vi "DataBuffer_NET-rebuild.VI"() -> ()   [LabVIEW 2016]
uses:
  C:/Program Files/Ocean Optics/OmniDriver/OOI_HOME/NETOmniDriver-NET20.dll
  Program Files/Ocean Optics/OmniDriver/OOI_HOME/NETOmniDriver-NET20.dll
panel:
  out "getBufferCapacity":i32
  out "isFeatureSupportedDataBuffer":i16
  in  "setBufferCapacity":i32
  in  "spectrometerIndex":i32
  out "Spectrometer Name:":string
  out "Serial Number:":string
  in  "Scans to Average":i32=1 min=1 max=50 step=1
  in  "Boxcar Width":i32=5 min=0 max=50 step=1
  in  "Int. Time (microsec)":i32=100000 min=3000 max=65000000
  out "Number of Spectrometers":i32
  in  "stop":bool
  out "Current Spectrum":cluster{"Y":dbl[], "Y":dbl[]}[](graph)
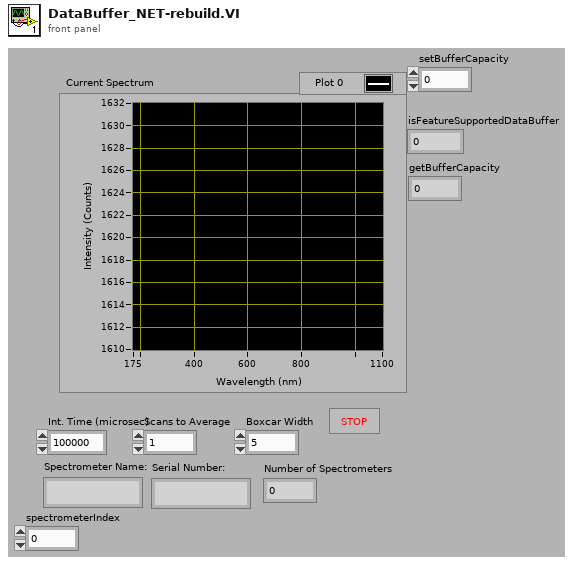
[diagram p1: front panel]
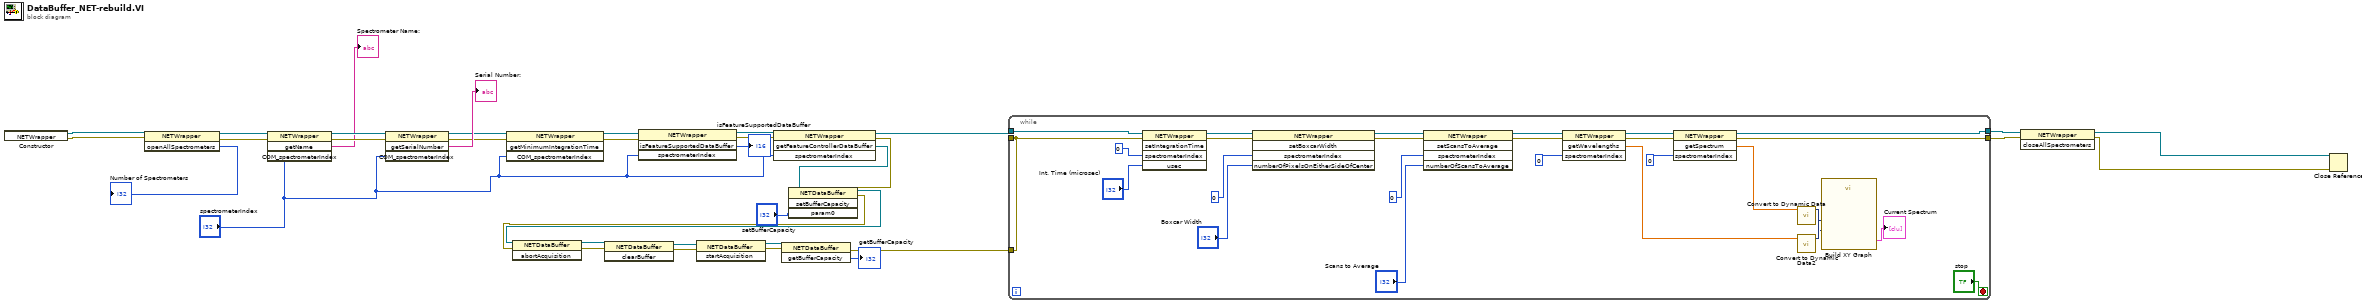
[diagram p0: block diagram]
diagram:
  n1 = constructor class="NETWrapper"() -> (reference out=w23:refnum<k24>, error out=w22:errorcluster)  [unwired: 3 in, 1 out]
  n2 = invoke class="NETWrapper" method="openAllSpectrometers"(reference=w23, error in=w22) -> (reference out=w31:refnum<k24>, error out=w30:errorcluster, "openAllSpectrometers"=→"Number of Spectrometers":i32)  [unwired: 1 in]
  n3 = invoke class="NETWrapper" method="getName"(reference=w31, error in=w30, "COM_spectrometerIndex"="spectrometerIndex") -> (reference out=w29:refnum<k24>, error out=w28:errorcluster, "getName"=→"Spectrometer Name:":string)  [unwired: 1 in, 1 out]
  n4 = invoke class="NETWrapper" method="getSerialNumber"(reference=w29, error in=w28, "COM_spectrometerIndex"="spectrometerIndex") -> (reference out=w26:refnum<k24>, error out=w25:errorcluster, "getSerialNumber"=→"Serial Number:":string)  [unwired: 1 in, 1 out]
  n5 = invoke class="NETWrapper" method="getMinimumIntegrationTime"(reference=w26, error in=w25, "COM_spectrometerIndex"="spectrometerIndex") -> (reference out=w21:refnum<k24>, error out=w20:errorcluster)  [unwired: 1 in, 2 out]
  n6 = invoke class="NETWrapper" method="isFeatureSupportedDataBuffer"(reference=w21, error in=w20, "spectrometerIndex"="spectrometerIndex") -> (reference out=w19:refnum<k24>, error out=w18:errorcluster, "isFeatureSupportedDataBuffer"=→"isFeatureSupportedDataBuffer":i16)  [unwired: 1 in, 1 out]
  n7 = invoke class="NETWrapper" method="getFeatureControllerDataBuffer"(reference=w19, error in=w18, "spectrometerIndex"="spectrometerIndex") -> (reference out=w17:refnum<k24>, error out=w9:errorcluster, "getFeatureControllerDataBuffer"=w11:refnum<k24>)  [unwired: 1 in, 1 out]
  n8 = invoke class="NETDataBuffer" method="setBufferCapacity"(reference=w11, error in=w9, "param0"="setBufferCapacity") -> (reference out=w10:refnum<k24>, error out=w7:errorcluster)  [unwired: 1 in, 2 out]
  n9 = invoke class="NETDataBuffer" method="abortAcquisition"(reference=w10, error in=w7) -> (reference out=w15:refnum<k24>, error out=w14:errorcluster)  [unwired: 1 in, 1 out]
  n10 = invoke class="NETDataBuffer" method="clearBuffer"(reference=w15, error in=w14) -> (reference out=w13:refnum<k24>, error out=w12:errorcluster)  [unwired: 1 in, 1 out]
  n11 = invoke class="NETDataBuffer" method="startAcquisition"(reference=w13, error in=w12) -> (reference out=w5:refnum<k24>, error out=w4:errorcluster)  [unwired: 1 in, 1 out]
  n12 = invoke class="NETDataBuffer" method="getBufferCapacity"(reference=w5, error in=w4) -> (error out=w8:errorcluster, "getBufferCapacity"=→"getBufferCapacity":i32)  [unwired: 1 in, 1 out]
  n13 = while {
    tunnel: [w58] -> w35
    tunnel: [w57] -> w34
    tunnel: w17 -> [w50]
    tunnel: [w36] -> _
    tunnel: w8 -> [w36]
    stop <- "stop" stop-if-true
    n14 = invoke class="NETWrapper" method="setIntegrationTime"(reference=w50, error in=w36, "spectrometerIndex"=0, "usec"="Int. Time (microsec)") -> (reference out=w47:refnum<k24>, error out=w46:errorcluster)  [unwired: 1 in, 3 out]
    n15 = invoke class="NETWrapper" method="setBoxcarWidth"(reference=w47, error in=w46, "spectrometerIndex"=0, "numberOfPixelsOnEitherSideOfCenter"="Boxcar Width") -> (reference out=w44:refnum<k24>, error out=w43:errorcluster)  [unwired: 1 in, 3 out]
    n16 = invoke class="NETWrapper" method="setScansToAverage"(reference=w44, error in=w43, "spectrometerIndex"=0, "numberOfScansToAverage"="Scans to Average") -> (reference out=w40:refnum<k24>, error out=w39:errorcluster)  [unwired: 1 in, 3 out]
    n17 = invoke class="NETWrapper" method="getWavelengths"(reference=w40, error in=w39, "spectrometerIndex"=0) -> (reference out=w60:refnum<k24>, error out=w59:errorcluster, "getWavelengths"=w37:dbl[])  [unwired: 1 in, 1 out]
    n18 = invoke class="NETWrapper" method="getSpectrum"(reference=w60, error in=w59, "spectrometerIndex"=0) -> (reference out=w57:refnum<k24>, error out=w58:errorcluster, "getSpectrum"=w38:dbl[])  [unwired: 1 in, 1 out]
    n19 = call "Convert to Dynamic Data"("Array"=w38) -> ("Dynamic Data Type"=w54:dynamicdata)  [unwired: 3 out]
    n20 = call "Convert to Dynamic Data2"("Array"=w37) -> ("Dynamic Data Type"=w55:dynamicdata)  [unwired: 3 out]
    n21 = call "Build XY Graph"("Y Input"=w54, "X Input"=w55) -> ("XY Graph"=→"Current Spectrum":cluster{"Y":dbl[], "Y":dbl[]}[])  [unwired: 3 in, 6 out]
  }
  n22 = invoke class="NETWrapper" method="closeAllSpectrometers"(reference=w34, error in=w35) -> (reference out=w2:refnum<k24>, error out=w24:errorcluster)  [unwired: 1 in, 1 out]
  n23 = Close Reference(reference=w2, error in (no error)=w24) -> ()  [unwired: 1 out]
